vi "ALTS-2015 Start Test.vi"(8 "error in (no error)":errorcluster, 11 "Station Cluster":T1) -> (0 "error out":errorcluster)   [LabVIEW 2013]
uses:
  Controls/ALTS-2015 Station Cluster.ctl
  Controls/ALTS-2015 DO Start Stop Options.ctl
  Controls/ALTS-2015 Digital Output Options.ctl
  Controls/ALTS-2015 LV2GBL Station Info Options.ctl
  Controls/ALTS-2015 Status Message Options.ctl
  Controls/ALTS-2015 Ring Indicator Enum.ctl
  Controls/ALTS-2015 Status Ring Indicator.ctl
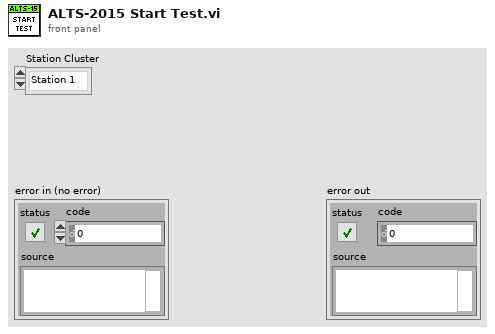
[diagram p1: front panel]
types:
  T1 = typedef "ALTS-2015 Station Cluster.ctl" = enum16{"Station 1", "Station 2", "Station 3", "Station 4"}
  T2 = typedef "ALTS-2015 LV2GBL Station Info Options.ctl" = enum16{"Init", "Read", "Read All", "Write Sensor ID", "Write  WO & SN", "Write Test Data", "Write Station Status", "Write Station Occupancy", "Write Rerun", "Clear All", "Clear Test Result"}
  T3 = typedef "ALTS-2015 Status Ring Indicator.ctl" = u16
  T4 = typedef "ALTS-2015 Ring Indicator Enum.ctl" = enum16{"Idle", "Test Running", "Unit Clamped", "Unit not Clamped", "Pass", "Fail"}
  T5 = typedef "ALTS-2015 Status Message Options.ctl" = enum16{"Initializing...", "Enter User Login...", "Enter Work Order Number...", "Enter Serial Number...", "Valid Serial Number...", "Invalid Serial Number...", "Start Tag Received...", "Stop Tag Received...", "UUT Clamped...", "UUT not Clamped...", "Test Running...", "Test Complete...", "Writing Result to DB...", "DB Entry Pressed...", "Clearing Serial Number...", "Idle...", "Exiting..."}
  T6 = typedef "ALTS-2015 Digital Output Options.ctl" = enum16{"Idle", "Test Running", "Pass", "Fail"}
  T7 = typedef "ALTS-2015 DO Start Stop Options.ctl" = enum16{"Start Test", "Stop Test"}
  T8 = typedef "ALTS-2015 Station Details.ctl" = cluster{"Station Number":string, "Work Order Number":string, "Sensor Name":string, "Pressure (PSI)":string, "Flow (SCCM)":string, "Test Time ":string, "Test Result":string, "Serial Number":string, "Station Status":T3, "Station Occupied?":bool, "Rerun Count":i32, "Test Type":i32}
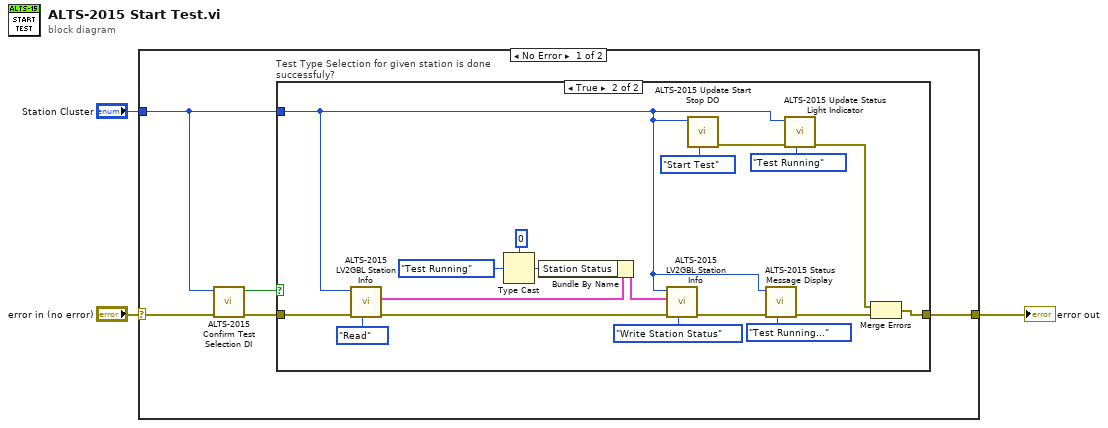
[diagram p0: block diagram]
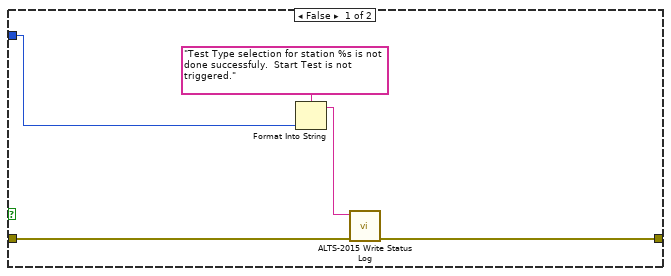
[diagram p2: hidden frame]
diagram:
  n1 = case shown="No Error" "error in (no error)" {
    selector: "error in (no error)" -> [w7 w32]
    tunnel: "Station Cluster" -> [w5 _]
    tunnel: [w8 w32] -> w2
    frame No Error {
      n2 = call "ALTS-2015 Confirm Test Selection DI.vi"("error in"=w7, "Station Cluster"=w5) -> ("error out"=w6:errorcluster, "Test Type Selection Successful"=w4:bool)  [unwired: 8 in]
      n3 = case "Test Type Selection for given station is done successfuly?" shown="True" w4 {
        tunnel: [w12 w25] -> w8
        tunnel: w5 -> [w11 w17]
        tunnel: w6 -> [w13 w16]
        frame False {
          n4 = Format Into String(format string="Test Type selection for station %s is not done successfuly.  Start Test is not triggered.", w11) -> (resulting string=w9:string)  [unwired: 2 in, 1 out]
          n5 = call "ALTS-2015 Write Status Log.vi"("error in (no error)"=w13, "Status Input"=w9) -> ("error out"=w12:errorcluster)  [unwired: 9 in]
        }
        frame True {
          n6 = call "ALTS-2015 LV2GBL Station Info.vi"("Options"=ALTS-2015_LV2GBL_Station_Info_Options."Read", "error in"=w16, "Station Cluster"=w17) -> ("error out"=w14:errorcluster, "Station Details"=w15:T8)  [unwired: 6 in, 1 out]
          n7 = Type Cast(type=T3 0 ("Station Status"), x=ALTS-2015_Ring_Indicator_Enum."Test Running" ("Ring Indicator Options")) -> (*(type *) &x=w20:T3)
          n8 = Bundle By Name(cluster=w15, "Station Status"=w20) -> (w19:T8)
          n9 = call "ALTS-2015 LV2GBL Station Info.vi"("Options"=ALTS-2015_LV2GBL_Station_Info_Options."Write Station Status", "error in"=w14, "Station"=w19, "Station Cluster"=w17) -> ("error out"=w27:errorcluster)  [unwired: 5 in, 2 out]
          n10 = call "ALTS-2015 Update Start Stop DO.vi"("DO Options"=ALTS-2015_DO_Start_Stop_Options."Start Test", "Station Cluster"=w17) -> ("error out"=w23:errorcluster)  [unwired: 9 in]
          n11 = call "ALTS-2015 Status Message Display.vi"("Status Message Options"=ALTS-2015_Status_Message_Options."Test Running...", "error in (no error)"=w27, "Station Enum"=w17) -> ("error out"=w31:errorcluster)  [unwired: 7 in, 1 out]
          n12 = call "ALTS-2015 Update Status Light Indicator.vi"("DO Options"=ALTS-2015_Digital_Output_Options."Test Running", "error in"=w23, "Station Cluster"=w17) -> ("error out"=w30:errorcluster)  [unwired: 8 in]
          n13 = Merge Errors(w30, w31) -> (w25:errorcluster)
        }
      }
    }
    frame Error {
    }
  }
  "error out" <- w2
